vi "read_raw_file.vi"() -> ()   [LabVIEW 2024]
panel:
  out "Reading":bool
  out "Num records":i32
  out "Timestamp":timestamp
  out "Record":i32
  in  "stop":bool
  in  "Scrollbar":i32(c297)
  out "Record size":i64
  in  "Card":i32=1
  out "Waveform Graph":waveform(dbl)[](graph)
  in  "Raw file":path
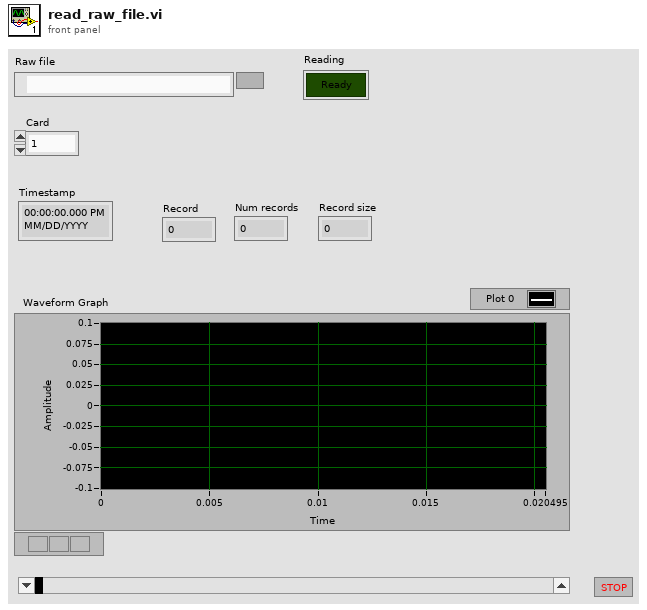
[diagram p1: front panel]
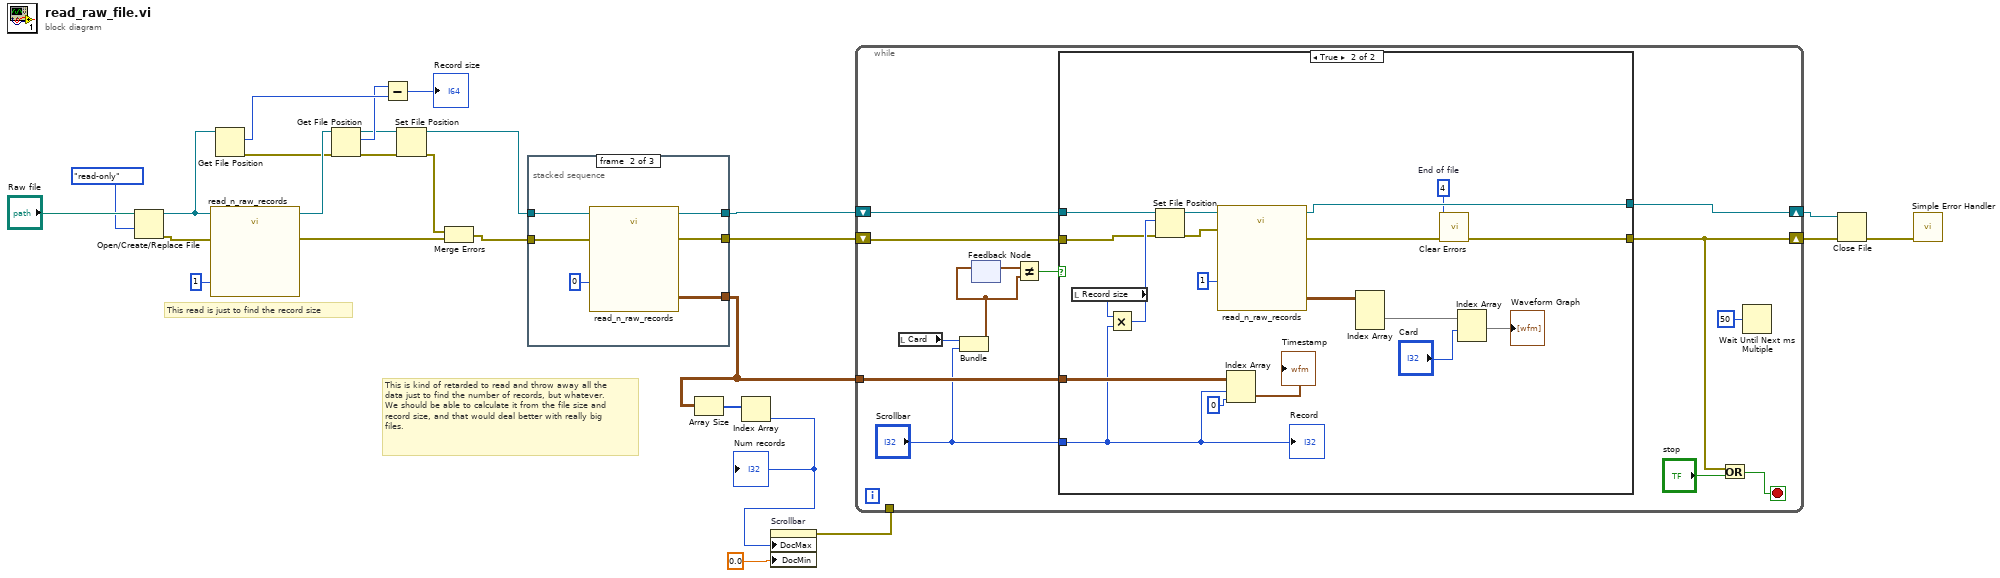
[diagram p0: block diagram]
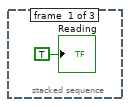
[diagram p2: hidden frame]
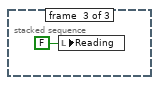
[diagram p3: hidden frame]
diagram:
  # "This is kind of retarded to read and throw away all the data just to find the number of records, but whatever. We should be able to calculate it from the file size and record size, and that would deal better with really big files."
  # "This read is just to find the record size"
  n1 = Open/Create/Replace File(file path (use dialog)="Raw file", access (0:read/write)=enum16{"read/write", "read-only", "write-only"}."read-only") -> (refnum out=w20:refnum<file>, error out=w24:errorcluster)  [unwired: 4 in, 1 out]
  n2 = call "read_n_raw_records.vi"("error in"=w24, "Num records"=1, "Byte Stream File in"=w20) -> ("error out"=w17:errorcluster, "Byte Stream File out"=w19:refnum<file>)  [unwired: 5 in, 2 out]
  n3 = Get File Position(7:w20) -> (0:w18:errorcluster, 2:w23:i64)  [unwired: 1 in, 1 out]
  n4 = Get File Position(4:w18, 7:w19) -> (0:w13:errorcluster, 2:w22:i64, 3:w14:refnum<file>)
  n5 = Subtract(x=w22, y=w23) -> (x-y=→"Record size":i64)
  n6 = Set File Position(refnum=w14, error in=w13) -> (refnum out=w11:refnum<file>, error out=w12:errorcluster)  [unwired: 2 in]
  n7 = Merge Errors(w12, w17) -> (w15:errorcluster)
  n8 = stacked-sequence {
    tunnel: w15 -> [_ w33 _]
    tunnel: [_ w31 _] -> w1
    tunnel: w11 -> [_ w30 _]
    tunnel: [_ w29 _] -> w10
    tunnel: [_ w28 _] -> w6
    frame #0 {
      "Reading" <- TRUE ("Reading")
    }
    frame #1 {
      n9 = call "read_n_raw_records.vi"("error in"=w33, "Num records"=0, "Byte Stream File in"=w30) -> ("error out"=w31:errorcluster, "Timestamps"=w28:timestamp[][], "Byte Stream File out"=w29:refnum<file>)  [unwired: 5 in, 1 out]
    }
    frame #2 {
      n10 = local write "Reading"(FALSE ("Reading")) -> ()
    }
  }
  n11 = Array Size(array=w6) -> (size(s)=w5:i32[])
  n12 = Index Array(array=w5) -> (element=w2:i32)  [unwired: 1 in]
  "Num records" <- w2
  n13 = property on="Scrollbar" class="Scroll (strict)"("DocMax"=w2, "DocMin"=0.0 ("Doc Min")) -> (error out=w3:errorcluster)  [unwired: 2 in, 1 out]
  n14 = while {
    tunnel: w6 -> [w46]
    shift-right: [w41] -> w9
    shift-left: w10 -> [w42]
    shift-right: [w40] -> w8
    shift-left: w1 -> [w43]
    tunnel: w3 -> [_]
    stop <- w38 stop-if-true
    n15 = local read "Card"() -> (w35:i32)
    n16 = Bundle("Card"=w35, "Scrollbar"="Scrollbar") -> (w37:cluster{"Card":i32, "Scrollbar":i32})  [unwired: 1 in]
    n17 = feedback-in #1(w37) -> ()
    n18 = feedback #1() -> (w45:cluster{"Card":i32, "Scrollbar":i32})  [unwired: 1 in]
    n19 = Not Equal?(x=w45, y=w37) -> (x != y?=w44:bool)
    n20 = case shown="True" w44 {
      tunnel: w46 -> [_ w68]
      tunnel: "Scrollbar" -> [_ w61]
      tunnel: w43 -> [w48 w58]
      tunnel: w42 -> [w49 w62]
      tunnel: [w48 w50] -> w40
      tunnel: [w49 w53] -> w41
      frame False {
      }
      frame True {
        w52 = 4  # End of file
        n21 = local read "Record size"() -> (w60:i64)
        n22 = Multiply(x=w60, y=w61) -> (x*y=w59:i64)
        n23 = Set File Position(offset (in bytes) (0)=w59, refnum=w62, error in=w58) -> (refnum out=w57:refnum<file>, error out=w54:errorcluster)  [unwired: 1 in]
        n24 = call "read_n_raw_records.vi"("error in"=w54, "Num records"=1, "Byte Stream File in"=w57) -> ("error out"=w51:errorcluster, "Input data"=w56:waveform(dbl)[][][], "Byte Stream File out"=w53:refnum<file>)  [unwired: 5 in, 1 out]
        n25 = Index Array(array=w68, index (row)=w61, index (col)=0 ("disabled index (col)")) -> (element=→"Timestamp":timestamp)
        n26 = Index Array(array=w56) -> (element=w55:waveform(dbl)[][])  [unwired: 3 in]
        n27 = call <vilib>:"Clear Errors.vi"("error in (no error)"=w51, "specific error code to clear (0: all)"=w52) -> ("error out"=w50:errorcluster)  [unwired: 4 in, 1 out]
        n28 = Index Array(array=w55, index (row)="Card") -> (element=→"Waveform Graph":waveform(dbl)[])  [unwired: 1 in]
        "Record" <- w61
      }
    }
    n29 = Or(x=w40, y="stop") -> (x .or. y?=w38:bool)
    n30 = Wait Until Next ms Multiple(millisecond multiple=u32 50) -> ()  [unwired: 1 out]
  }
  n31 = Close File(refnum=w9, error in=w8) -> (error out=w7:errorcluster)  [unwired: 1 out]
  n32 = call <vilib>:"Simple Error Handler.vi"("error in (no error)"=w7) -> ()  [unwired: 4 in, 5 out]
